vi "AnalogOutput.vi"(7 "Read or Set Voltage?":enum16{"Read Voltage", "Set Voltage"}(ring)=enum."Set Voltage", 8 "Voltage Safety Limit":dbl=10.0, 9 "Increment":dbl=0.1, 10 "Target Voltage":dbl, 11 "Channel":T1(ring)=enum."Output 3 (V)") -> (3 "Output Voltage":sgl format="%#_8p")   [LabVIEW 2021]
uses:
  <userlib>/Nanonis Prog Interface V5/Nanonis Prog Interface.lvlib
panel:
  in  "milliseconds to wait":u32=50
  in  "Stop":bool
  # "Analog Output Increment"
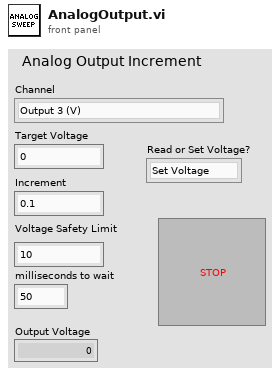
[diagram p1: front panel]
types:
  T1 = enum16{"Output 2 (V)", "Output 3 (V)", "Output 4 (V)"}
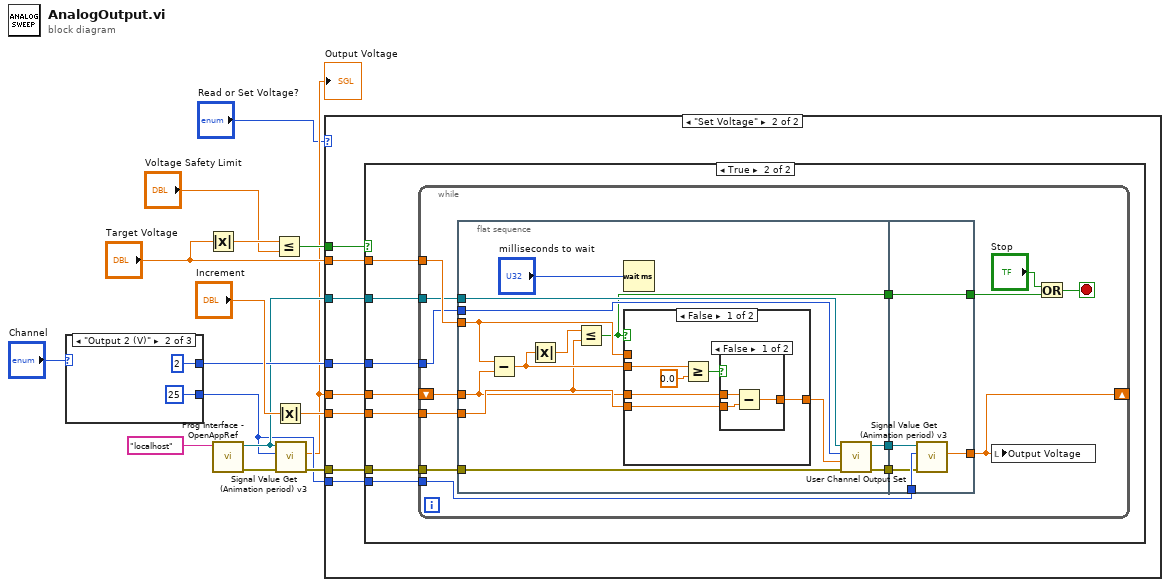
[diagram p0: block diagram]
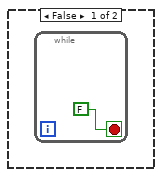
[diagram p3: hidden frame]
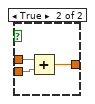
[diagram p4: hidden frame]
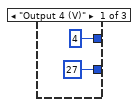
[diagram p6: hidden frame]
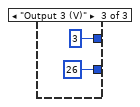
[diagram p7: hidden frame]
diagram:
  n1 = case shown="\"Output 2 (V)\"" "Channel" {
    tunnel: [i8 27 ("Signal index (0-127)") i8 25 ("Signal index (0-127)") i8 26 ("Signal index (0-127)")] -> w3
    tunnel: [u8 4 ("User output channel") u8 2 ("User output channel") u8 3 ("User output channel")] -> w6
    frame "Output 4 (V)" {
    }
    frame "Output 2 (V)" {
    }
    frame "Output 3 (V)" {
    }
  }
  n2 = Absolute Value(x="Target Voltage") -> (abs(x)=w11:dbl)
  n3 = call <userlib>:"Prog Interface - OpenAppRef.vi"("Machine name (local machine IP)"="localhost" ("machine name (localhost)")) -> ("Error out"=w13:errorcluster, "Application reference"=w5:refnum<vi>)  [unwired: 5 in]
  n4 = Less Or Equal?(x=w11, y="Voltage Safety Limit") -> (x <= y?=w10:bool)
  n5 = Absolute Value(x="Increment") -> (abs(x)=w12:dbl)
  n6 = call <userlib>:"Signal Value Get (Animation period) v3.vi"("error in (no error)"=w13, "Signal index (0-127)"=w3, "Application ref in"=w5) -> ("error out"=w4:errorcluster, "Signal value"=w2:sgl)  [unwired: 5 in, 1 out]
  "Output Voltage" <- w2
  n7 = case shown="\"Set Voltage\"" "Read or Set Voltage?" {
    tunnel: w12 -> [_ w29]
    tunnel: w10 -> [_ w28]
    tunnel: "Target Voltage" -> [_ w27]
    tunnel: w6 -> [_ w26]
    tunnel: w5 -> [_ w25]
    tunnel: w4 -> [_ w24]
    tunnel: w3 -> [_ w23]
    tunnel: w2 -> [_ w22]
    frame "Read Voltage", Default {
    }
    frame "Set Voltage" {
      n8 = case shown="True" w28 {
        tunnel: w27 -> [_ w37]
        tunnel: w22 -> [_ w32]
        tunnel: w29 -> [_ w36]
        tunnel: w26 -> [_ w35]
        tunnel: w25 -> [_ w34]
        tunnel: w24 -> [_ w33]
        tunnel: w23 -> [_ w31]
        frame False {
          n9 = while {
            stop <- FALSE stop-if-true
          }
        }
        frame True {
          n10 = while {
            tunnel: w37 -> [w50]
            tunnel: w36 -> [w51]
            shift-right: [w40] -> _
            shift-left: w32 -> [w49]
            tunnel: w35 -> [w48]
            tunnel: w34 -> [w47]
            tunnel: w33 -> [w46]
            tunnel: w31 -> [w45]
            stop <- w42 stop-if-true
            n11 = flat-sequence {
              tunnel: w50 -> [w63]
              tunnel: w51 -> [w61]
              tunnel: w49 -> [w60]
              tunnel: w48 -> [w58]
              tunnel: w47 -> [w57]
              tunnel: w46 -> [w56]
              tunnel: [w55] -> w44
              tunnel: [w54] -> w43
              tunnel: [w52] -> w39
              tunnel: [w79] -> w40
              tunnel: w45 -> [w82]
              tunnel: w44 -> [w81]
              tunnel: w43 -> [w80]
              tunnel: [w78] -> w38
              tunnel: w39 -> [w78]
              frame #0 {
                n12 = Subtract(x=w63, y=w60) -> (x-y=w62:dbl)
                n13 = Absolute Value(x=w62) -> (abs(x)=w64:dbl)
                n14 = Less Or Equal?(x=w64, y=w61) -> (x <= y?=w52:bool)
                n15 = Wait (ms)(milliseconds to wait="milliseconds to wait") -> ()  [unwired: 1 out]
                n16 = case shown="False" w52 {
                  tunnel: w63 -> [_ w77]
                  tunnel: w62 -> [w67 _]
                  tunnel: w61 -> [w70 _]
                  tunnel: w60 -> [w66 _]
                  tunnel: [w65 w77] -> w59
                  frame False {
                    n17 = Greater Or Equal?(x=w67, y=0.0) -> (x >= y?=w69:bool)
                    n18 = case shown="False" w69 {
                      tunnel: w70 -> [w73 w76]
                      tunnel: w66 -> [w72 w75]
                      tunnel: [w71 w74] -> w65
                      frame False {
                        n19 = Subtract(x=w72, y=w73) -> (x-y=w71:dbl)
                      }
                      frame True {
                        n20 = Add(x=w75, y=w76) -> (x+y=w74:dbl)
                      }
                    }
                  }
                  frame True {
                  }
                }
                n21 = call <userlib>:"User Channel Output Set.vi"("error in (no error)"=w56, "Output value (physical unit)"=w59, "User output channel"=w58, "Application ref in"=w57) -> ("error out"=w54:errorcluster, "Application ref out"=w55:refnum<vi>)  [unwired: 5 in]
              }
              frame #1 {
                n22 = call <userlib>:"Signal Value Get (Animation period) v3.vi"("error in (no error)"=w80, "Signal index (0-127)"=w82, "Application ref in"=w81) -> ("Signal value"=w79:sgl)  [unwired: 5 in, 2 out]
              }
            }
            n23 = local write "Output Voltage"(w40) -> ()
            n24 = Or(x="Stop", y=w38) -> (x .or. y?=w42:bool)
          }
        }
      }
    }
  }
